vi "PID tester gyro.vi"   [LabVIEW 2016]
types:
  T1 = typedef "LVHSConnector.ctl" = refnum<class "BrickReference.lvclass">
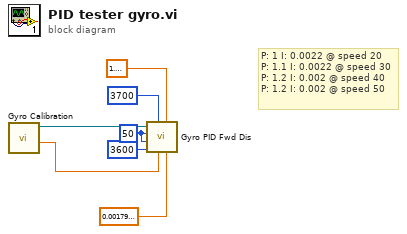
[diagram p0: block diagram]
diagram:
  w1 = 50 ("Max. speed")
  # "P: 1 I: 0.0022 @ speed 20\nP: 1.1 I: 0.0022 @ speed 30\nP: 1.2 I: 0.002 @ speed 40\nP: 1.2 I: 0.002 @ speed 50"
  n1 = call "Gyro Calibration.vi"() -> ("Degrees"=w5:sgl, "NXT/EV3"=w6:T1)  [unwired: 7 in, 1 out]
  n2 = call "Gyro PID Fwd Dis.vi"("K_i"=sgl 0.0018, "K_p"=sgl 1.3, "Target angle"=w5, "Threshold to stop"=3700, "Threshold to slow"=3600, "Min. speed"=w1, "Max. speed"=w1, "EV3 in"=w6) -> ()  [unwired: 3 in, 1 out]
